vi "Measure.vi"(0 "Keysight_34401A-DMM in":refnum<class "Keysight_34401A-DMM.lvclass">, 5 "Measure_Parameters":variant, 11 "error in (no error)":errorcluster) -> (4 "Keysight_34401A-DMM out":refnum<class "Keysight_34401A-DMM.lvclass">, 6 "Measure_Results":variant, 15 "error out":errorcluster)   [LabVIEW 2020, in "Abstract_Instrument.lvlib" / "Keysight_34401A-DMM.lvclass"]
uses:
  Keysight_34401A-DMM.lvclass
  <instrlib>/Agilent 34401/Public/Data/Read (Single Point).vi
  <instrlib>/Agilent 34401/Agilent 34401.lvlib
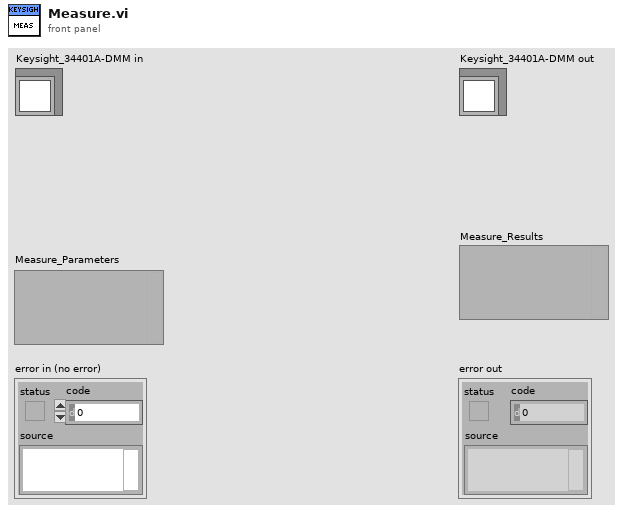
[diagram p1: front panel]
types:
  T1 = typedef "Abstract_Instrument.lvlib/Keysight_34401A-DMM.lvclass/Connection with Session.ctl" = cluster{"connection":T2, "session":refnum<visa-resource-name>}
  T2 = typedef "MeasurementLink Session Management V1.lvlib/Session Reservation.lvclass/Connection.ctl" = cluster{"pin or relay name":string, "site":i32, "instrument type id":string, "channel":string}
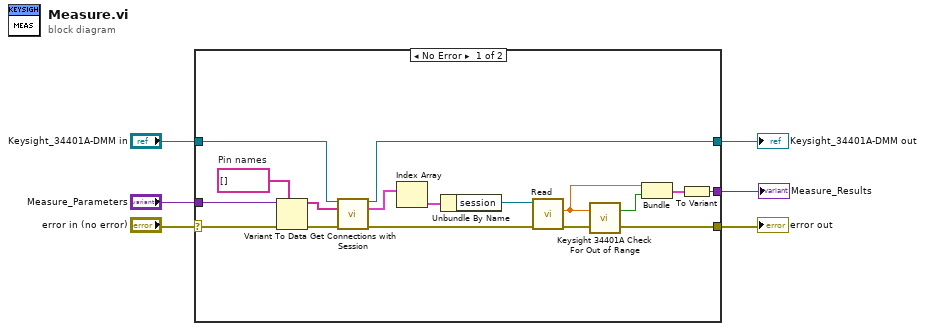
[diagram p0: block diagram]
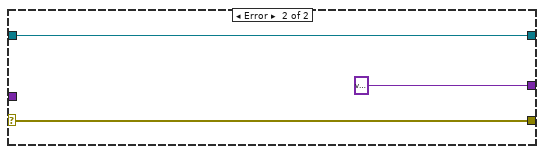
[diagram p2: hidden frame]
diagram:
  n1 = case shown="No Error" "error in (no error)" {
    selector: "error in (no error)" -> [w22 w23]
    tunnel: [w21 w23] -> w5
    tunnel: "Keysight_34401A-DMM in" -> [w12 w25]
    tunnel: [w17 variant ("Variant")] -> w3
    tunnel: [w13 w25] -> w2
    tunnel: "Measure_Parameters" -> [w16 _]
    frame No Error {
      w15 = string[] []  # Pin names
      n2 = Variant To Data(error in=w22, type=w15, Variant=w16) -> (data=w14:string[], error out=w11:errorcluster)
      n3 = call "Get Connections with Session.vi"("Keysight_34401A-DMM in"=w12, "pin or relay names"=w14, "error in (no error)"=w11) -> ("Keysight_34401A-DMM out"=w13:refnum<class "Keysight_34401A-DMM.lvclass">, "connections"=w9:T1[], "error out"=w10:errorcluster)  [unwired: 10 in]
      n4 = Index Array(array=w9) -> (element=w8:T1)  [unwired: 1 in]
      n5 = Unbundle By Name(w8) -> ("session"=w7:refnum<visa-resource-name>)
      n6 = call-poly <instrlib>:"Read.vi"("error in (no error)"=w10, "VISA resource name"=w7) -> ("error out"=w21:errorcluster, "Measurement"=w20:dbl)  [unwired: 7 in, 1 out]
      n7 = call "Keysight 34401A Check For Out of Range.vi"("value"=w20) -> ("out of range?"=w19:bool)  [unwired: 2 in]
      n8 = Bundle("Measurement"=w20, "out of range?"=w19) -> (w18:cluster{"Measurement":dbl, "out of range?":bool})  [unwired: 1 in]
      n9 = To Variant(anything=w18) -> (Variant=w17:variant)
    }
    frame Error {
    }
  }
  "error out" <- w5
  "Keysight_34401A-DMM out" <- w2
  "Measure_Results" <- w3
